vi "EncodeAddress.vi"(7 "AddressType":T1, 10 "Address":u16 max=16383) -> (2 "PololuAddressString":string)   [LabVIEW 2018]
uses:
  TicAddressStyle.ctl
panel:
  out "16bits":bool[](array[boolean])
  out "hexBytes":u32[](array[numeric]) format="%02x"
  out "individualBytes":bool[][](array[boolean])
  # "\"By default, these device numbers must be between 0 and 127, but with this new release you can enable 14-bit device numbers, which extends both device numbers so they can be any number from 0 to 16383.  In that case, the Tic will expect two device number bytes in every Pololu protocol command: the first device number byte holds bits 0 through 6 of the device number, while the second device number byte holds bits 7 through 13.\"\n-Jan Malasek (Pololu) 25-May-2018"
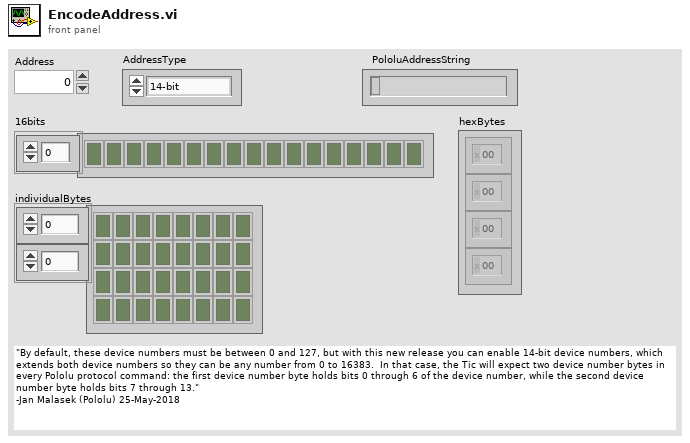
[diagram p1: front panel]
types:
  T1 = typedef "TicAddressStyle.ctl" = enum16{"14-bit", "7-bit"}
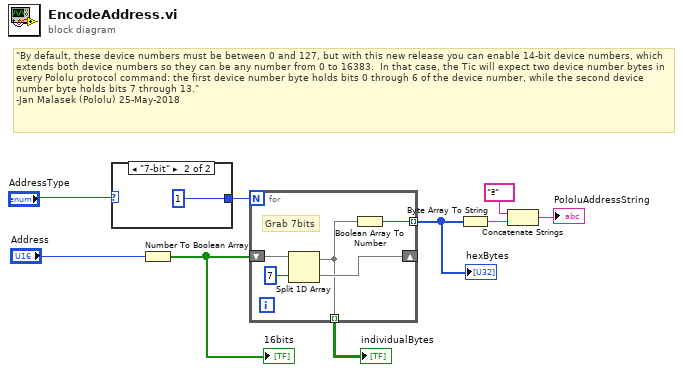
[diagram p0: block diagram]
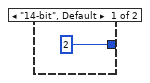
[diagram p2: hidden frame]
diagram:
  # "\"By default, these device numbers must be between 0 and 127, but with this new release you can enable 14-bit device numbers, which extends both device numbers so they can be any number from 0 to 16383.  In that case, the Tic will expect two device number bytes in every Pololu protocol command: the first device number byte holds bits 0 through 6 of the device number, while the second device number byte holds bits 7 through 13.\"\n-Jan Malasek (Pololu) 25-May-2018"
  n1 = case shown="\"7-bit\"" "AddressType" {
    tunnel: [2 1] -> w8
    frame "14-bit", Default {
    }
    frame "7-bit" {
    }
  }
  n2 = Number To Boolean Array(number="Address") -> (Boolean array=w7:bool[])
  "16bits" <- w7
  n3 = for {
    N: w8 -> [_]
    shift-right: [w15] -> _
    shift-left: w7 -> [w13]
    tunnel: [w14] -> w5 mode=indexing
    tunnel: [w12] -> w9 mode=indexing
    # "Grab 7bits"
    n4 = Split 1D Array(array=w13, index=7 ("length")) -> (first subarray=w12:bool[], second subarray=w15:bool[])
    n5 = Boolean Array To Number(Boolean array=w12) -> (number=w14:u32)
  }
  "hexBytes" <- w5
  "individualBytes" <- w9
  n6 = Byte Array To String(unsigned byte array=w5) -> (string=w3:string)
  n7 = Concatenate Strings("ª", w3) -> (→"PololuAddressString":string)
